vi "Eventos2.vi"() -> ()   [LabVIEW 2018]
uses:
  <vilib>/RAFA Solutions/Harmony UI Controls Kit/List, Table & Tree/Multicolumn Listbox.ctl
  <vilib>/RAFA Solutions/Harmony UI Controls Kit/Flat UI Design.lvlib
panel:
  in  "Tabla Eventos":T1
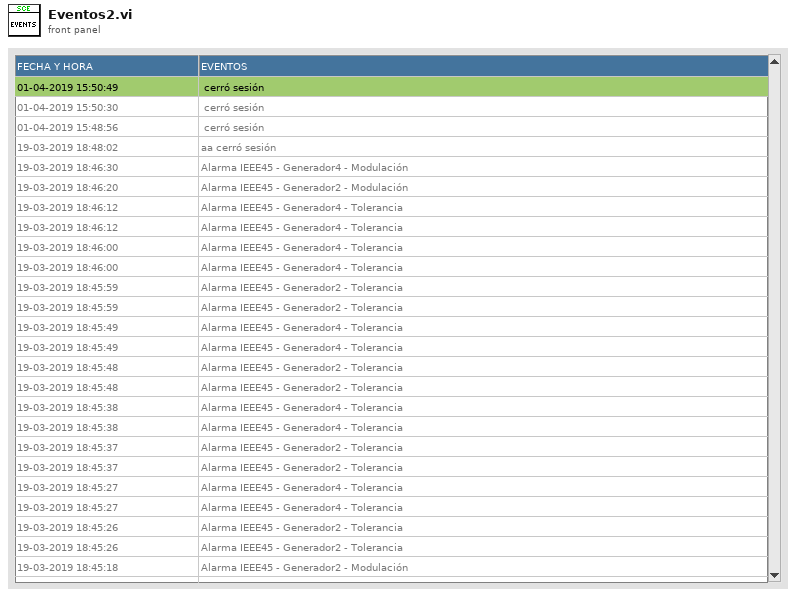
[diagram p1: front panel]
types:
  T1 = typedef "Flat UI Design.lvlib/Multicolumn Listbox.ctl" = i32
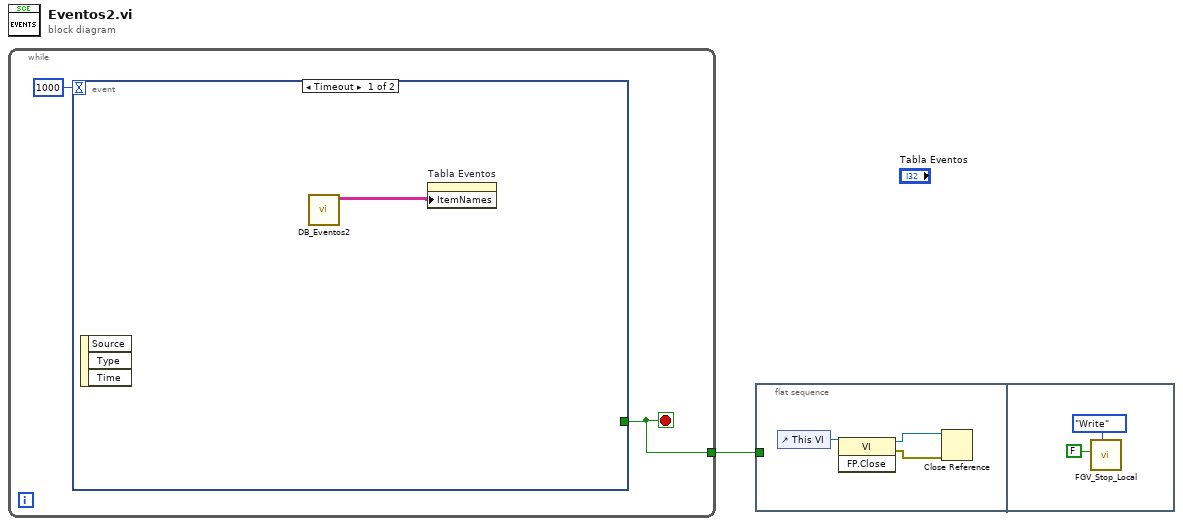
[diagram p0: block diagram]
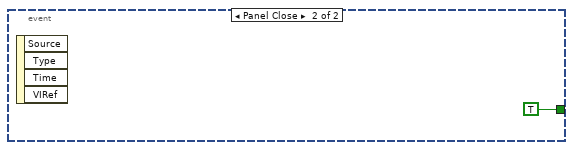
[diagram p2: hidden frame]
diagram:
  n1 = while {
    tunnel: [w3] -> w1
    stop <- w3 stop-if-true
    n2 = event shown="[0] Timeout" {
      selector: _ -> [_ _]
      dyn-events: _ -> [_ _]
      timeout: 1000 -> [_ _]
      tunnel: [_ TRUE] -> w3
      event Timeout {
        n3 = event-data() -> ()  [unwired: 1 in, 3 out]
        n4 = call "DB_Eventos2.vi"() -> ("Data"=w4:string[][])  [unwired: 10 in, 1 out]
        n5 = property on="Tabla Eventos" class="MCListbox (strict)"("ItemNames"=w4) -> ()  [unwired: 2 in, 2 out]
      }
      event Panel Close {
        n6 = event-data() -> ()  [unwired: 1 in, 4 out]
      }
    }
  }
  n7 = flat-sequence {
    tunnel: w1 -> [_]
    frame #0 {
      n8 = control-ref of="This VI"() -> (w8:refnum<vi>)
      n9 = invoke class="VI" method="FP.Close"(reference=w8) -> (reference out=w7:refnum<vi>, error out=w6:errorcluster)  [unwired: 2 in, 1 out]
      n10 = Close Reference(reference=w7, error in (no error)=w6) -> ()  [unwired: 1 out]
    }
    frame #1 {
      n11 = call "FGV_Stop_Local.vi"("Action"=enum16{"Read", "Write"}."Write", "Var In"=FALSE) -> ()  [unwired: 8 in, 2 out]
    }
  }
